vi "Sigma1.vi"(1 "e":u32) -> (0 "S1":u32)   [LabVIEW 2019]
doc: "Calculates the S1 variable for the compression phase"
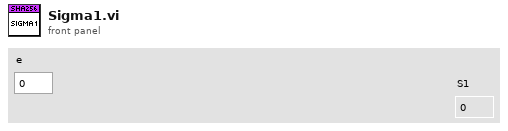
[diagram p1: front panel]
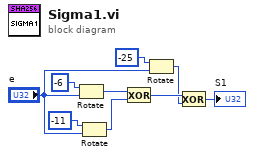
[diagram p0: block diagram]
diagram:
  n1 = Rotate(1:"e", 2:i16 -6 ("y")) -> (0:w5:u32)
  n2 = Rotate(1:"e", 2:i16 -11 ("y")) -> (0:w4:u32)
  n3 = Exclusive Or(1:w4, 2:w5) -> (0:w3:u32)
  n4 = Rotate(1:"e", 2:i16 -25 ("y")) -> (0:w2:u32)
  n5 = Exclusive Or(1:w2, 2:w3) -> (0:→"S1":u32)
